vi "2D Gaussian Kernel.vi"(9 "Standard Deviation":dbl=1.0, 10 "Gaussian Kernel Y Dimension":i32=11, 11 "Gaussian Kernel X Dimension":i32=11) -> (3 "Kernel":dbl[][](graph))   [LabVIEW 2011]
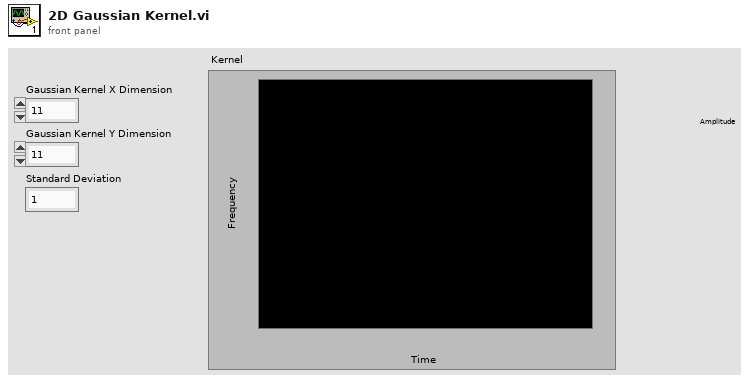
[diagram p1: front panel]
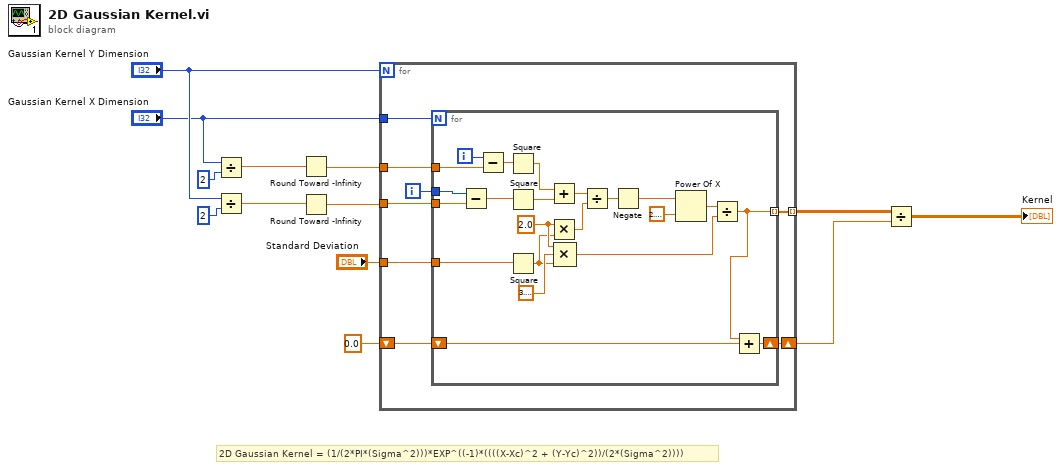
[diagram p0: block diagram]
diagram:
  # "2D Gaussian Kernel = (1/(2*PI*(Sigma^2)))*EXP^((-1)*((((X-Xc)^2 + (Y-Yc)^2))/(2*(Sigma^2))))"
  n1 = Divide(x="Gaussian Kernel X Dimension", y=2) -> (x/y=w7:dbl)
  n2 = Divide(x="Gaussian Kernel Y Dimension", y=2) -> (x/y=w6:dbl)
  n3 = Round Toward -Infinity(1:w7) -> (0:w8:dbl)
  n4 = Round Toward -Infinity(1:w6) -> (0:w5:dbl)
  n5 = for {
    N: "Gaussian Kernel Y Dimension" -> [_]
    tunnel: "Standard Deviation" -> [w21]
    tunnel: w5 -> [w20]
    tunnel: w8 -> [w19]
    tunnel: "Gaussian Kernel X Dimension" -> [w18]
    tunnel: [w17] -> w3 mode=indexing
    shift-right: [w14] -> w1
    shift-left: 0.0 -> [w15]
    i -> [w16]
    n6 = for {
      N: w18 -> [_]
      tunnel: w21 -> [w34]
      tunnel: w20 -> [w30]
      tunnel: w19 -> [w29]
      tunnel: [w24] -> w17 mode=indexing
      tunnel: w16 -> [w27]
      shift-right: [w22] -> w14
      shift-left: w15 -> [w23]
      i -> [w28]
      w35 = 2.0 ("x")
      n7 = Subtract(x=w27, y=w30) -> (x-y=w31:dbl)
      n8 = Subtract(x=w28, y=w29) -> (x-y=w32:dbl)
      n9 = Square(x=w32) -> (x^2=w39:dbl)
      n10 = Square(x=w31) -> (x^2=w38:dbl)
      n11 = Square(x=w34) -> (x^2=w25:dbl)
      n12 = Add(x=w39, y=w38) -> (x+y=w42:dbl)
      n13 = Multiply(x=w35, y=w25) -> (x*y=w26:dbl)
      n14 = Compound Arithmetic op=MULTIPLY(w35, 3.141592653589793, w25) -> (w33:dbl)
      n15 = Divide(x=w42, y=w26) -> (x/y=w40:dbl)
      n16 = Negate(x=w40) -> (-x=w41:dbl)
      n17 = Power Of X(1:2.718281828459045, 2:w41) -> (0:w37:dbl)
      n18 = Divide(x=w37, y=w33) -> (x/y=w24:dbl)
      n19 = Add(x=w24, y=w23) -> (x+y=w22:dbl)
    }
  }
  n20 = Divide(x=w3, y=w1) -> (x/y=→"Kernel":dbl[][])
